vi "Main.vi"() -> ()   [LabVIEW 2021]
doc: "Use this template to build a simple state machine design pattern. Each state executes code and determines which state to transition to."
uses:
  controls/State.ctl
  controls/Data.ctl
  vmmultmso/vmmultmso.lvlib
panel:
  out "Device is OK?":bool
  out "Sample Rate 2":dbl
  out "Voltage Wave":dbl[][](graph)
  out "Device2 ID":dbl
  out "Sample Rate":dbl
  out "Device1 ID":dbl
  out "CH2 Min":dbl
  out "CH2 Max":dbl
  out "CH2 Vpp":dbl
  out "CH2 Frequency":dbl
  out "CH1 Frequency":dbl
  out "CH1 Vpp":dbl
  out "CH1 Max":dbl
  out "CH1 Min":dbl
  out "IO Read Return":u32 format="%x"
  out "IO4":bool
  out "IO0":bool
  out "Is IO Ready?":bool
  in  "DDS2 Amplitude":dbl=2000.0
  in  "DDS2 Bias":dbl
  in  "DDS2 Freq":dbl=1000.0
  in  "DDS2 Wave Style":u16(ring) items=["Sine", "Square", "Ramp"]
  in  "DDS1 Amplitude":dbl=2000.0
  in  "DDS1 Bias":dbl
  in  "DDS1 Freq":dbl=1000.0
  in  "DDS1 Wave Style":u16(ring) items=["Sine", "Square", "Ramp"]
  out "Is Data Ready？":bool
  out "ReadVoltageData Return":u32
  out "Voltage Wave":dbl[][](graph)
  out "Capture Return":i32
  out "Support Samples":u32[](array[numeric])
  in  "Exit":bool
  # "DDS1"
  # "DDS2"
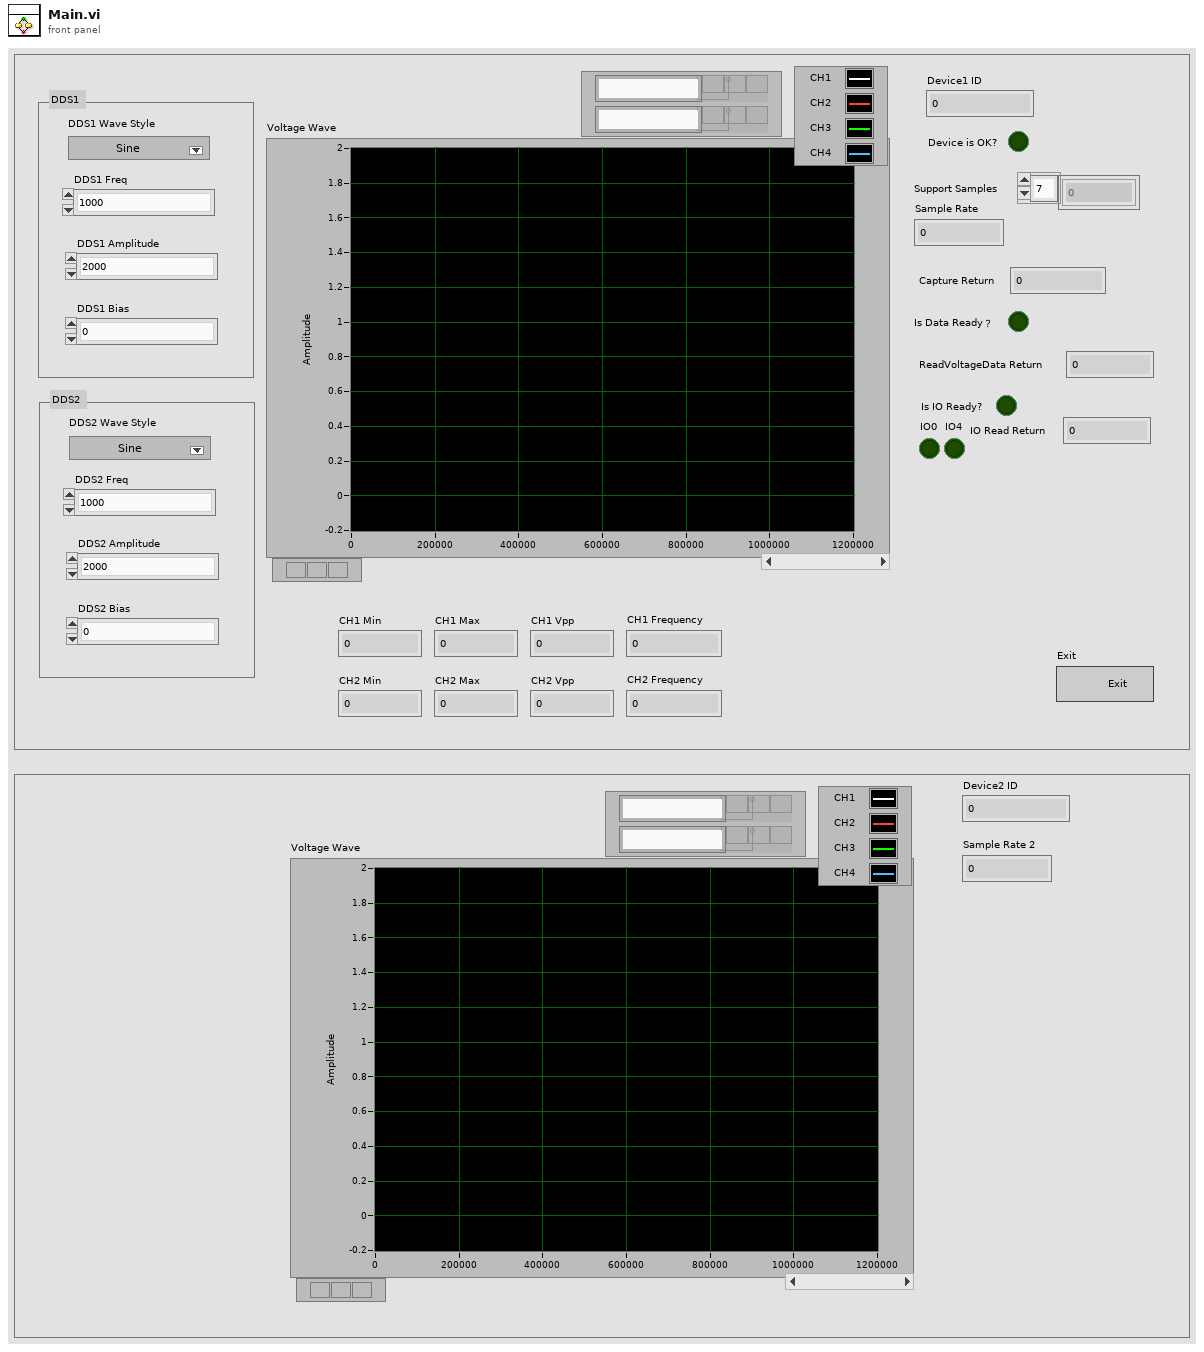
[diagram p1: front panel]
types:
  T1 = typedef "Data.ctl" = cluster{"Boolean <Is Exit>":bool, "String <Replace Me>":string, "Captue Length":dbl, "Device1 ID":dbl, "Device2 ID":dbl}
  T2 = typedef "State.ctl" = enum16{"Initialize", "Wait for UsbIn", "Init Osc and Dds", "Wait for Event", "Capture", "Read Voltage", "Read IO", "Exit"}
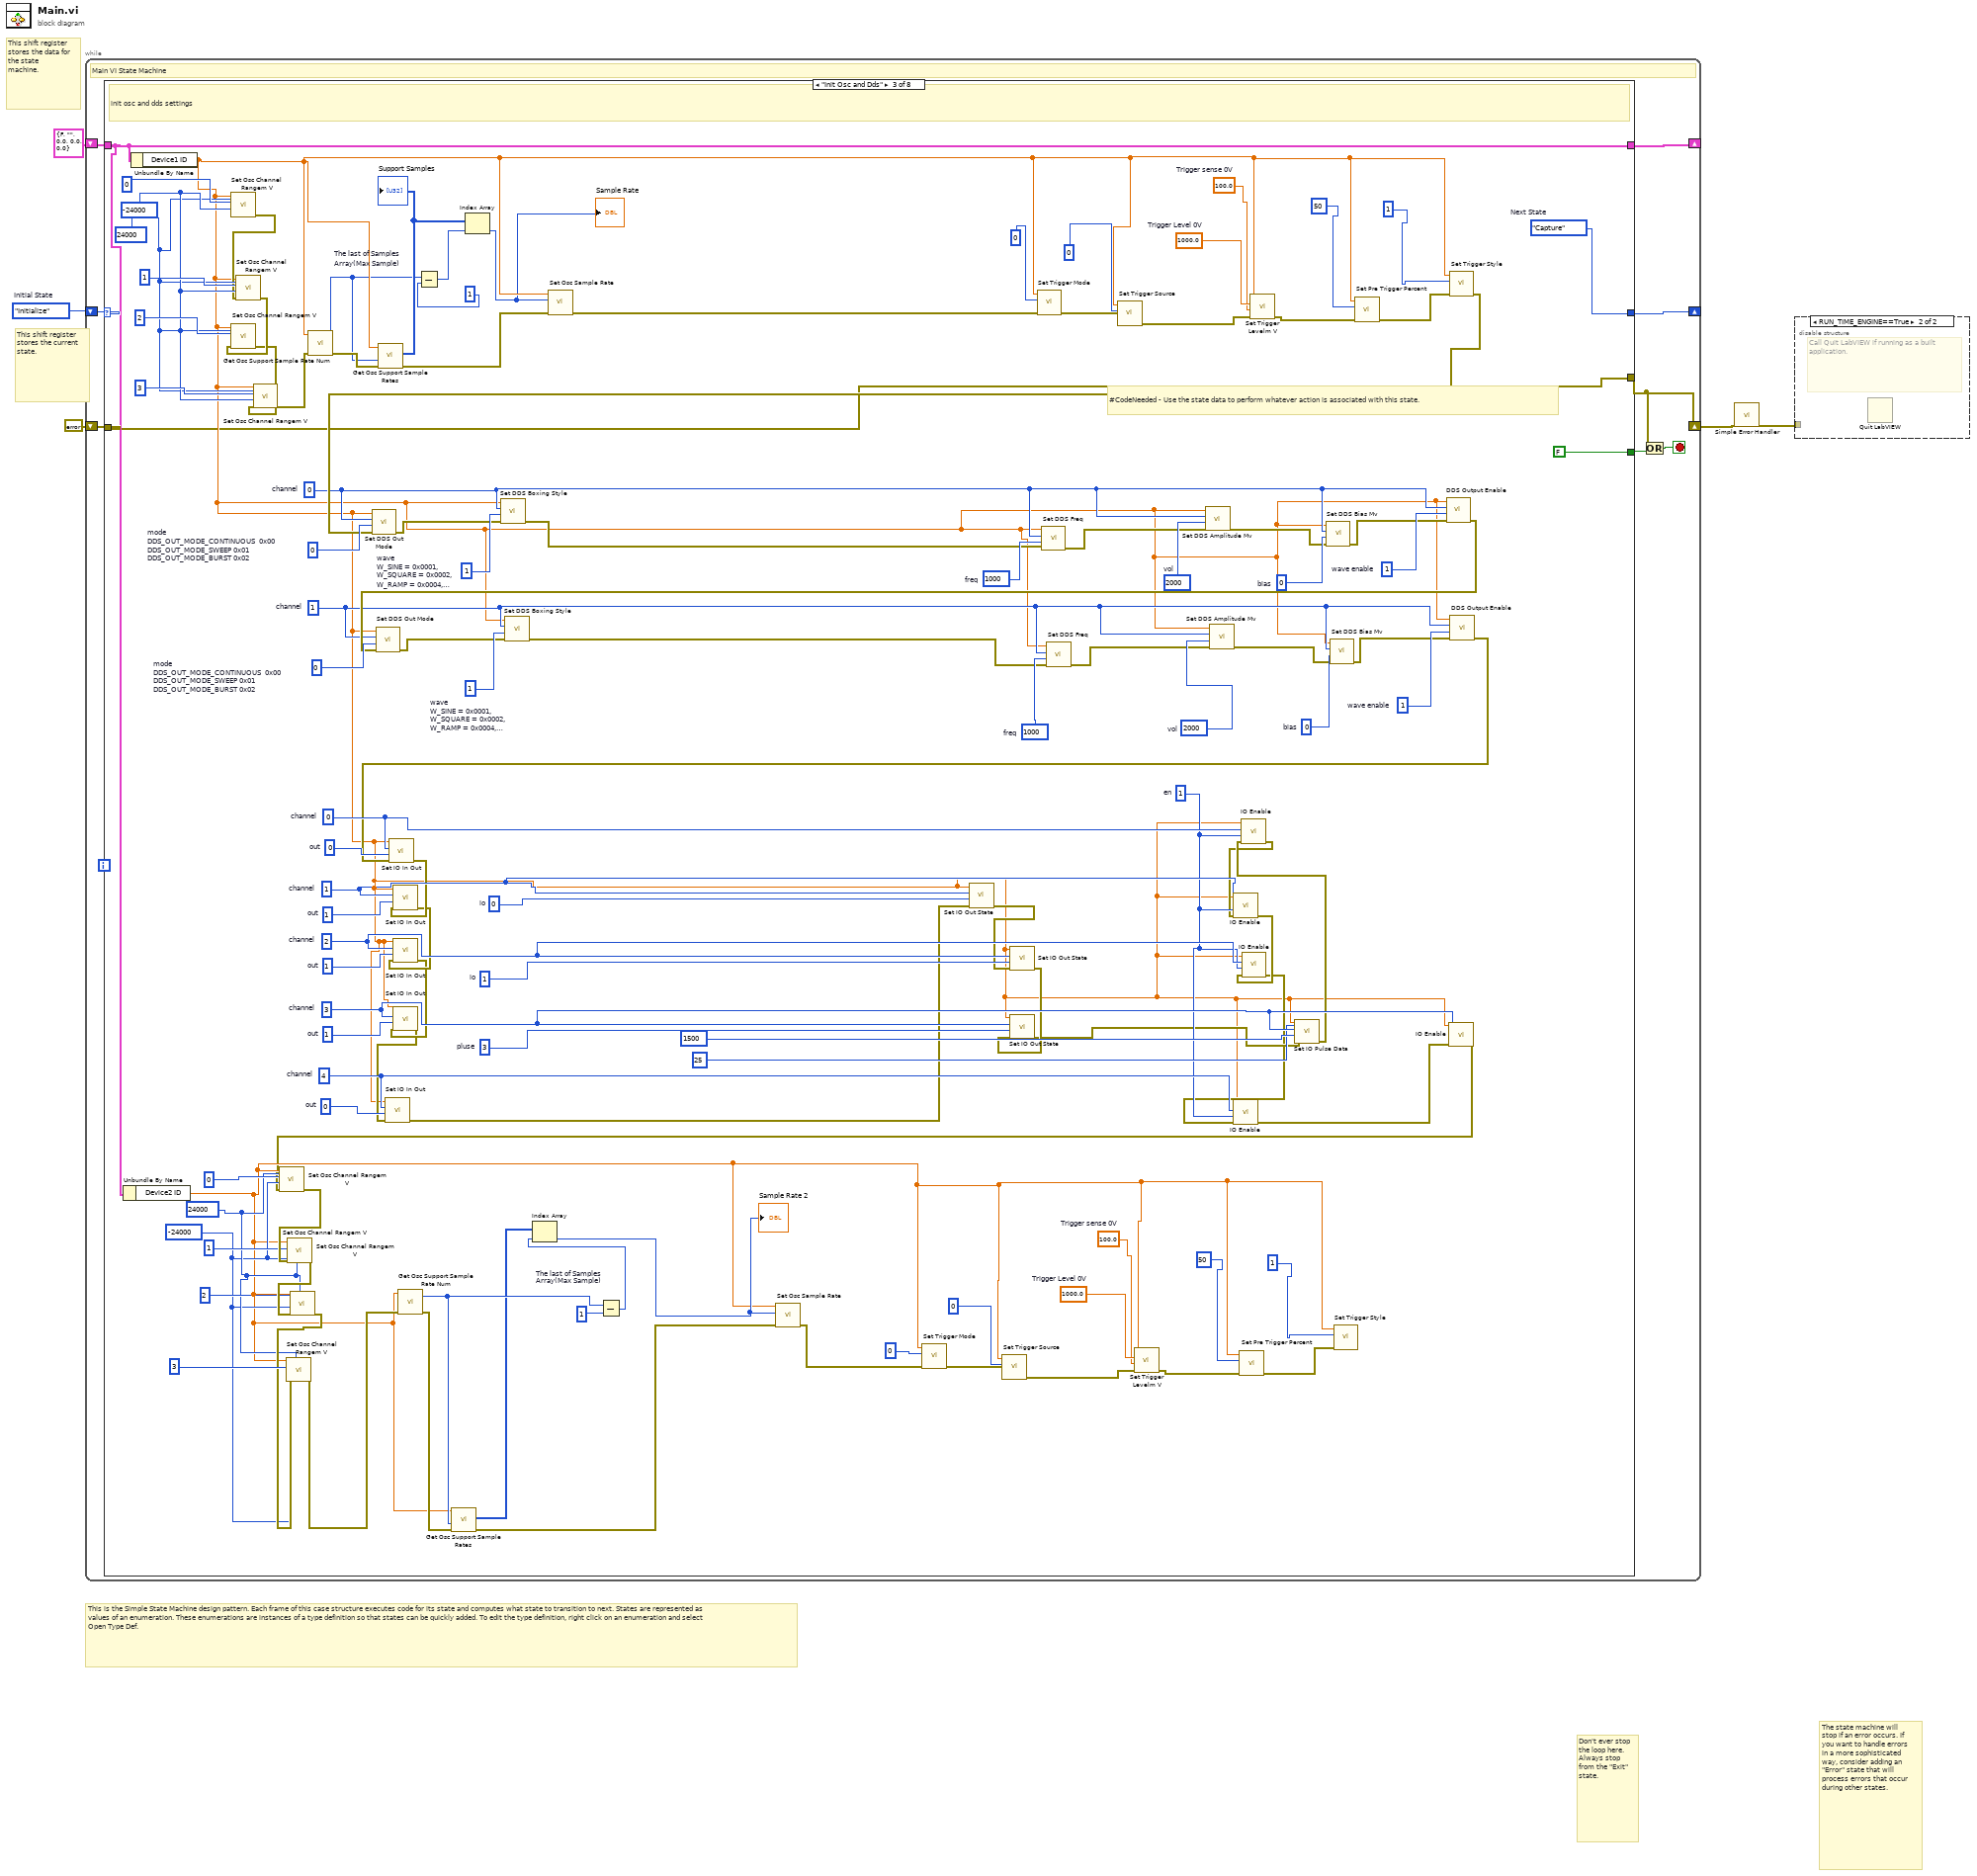
[diagram p0: block diagram]
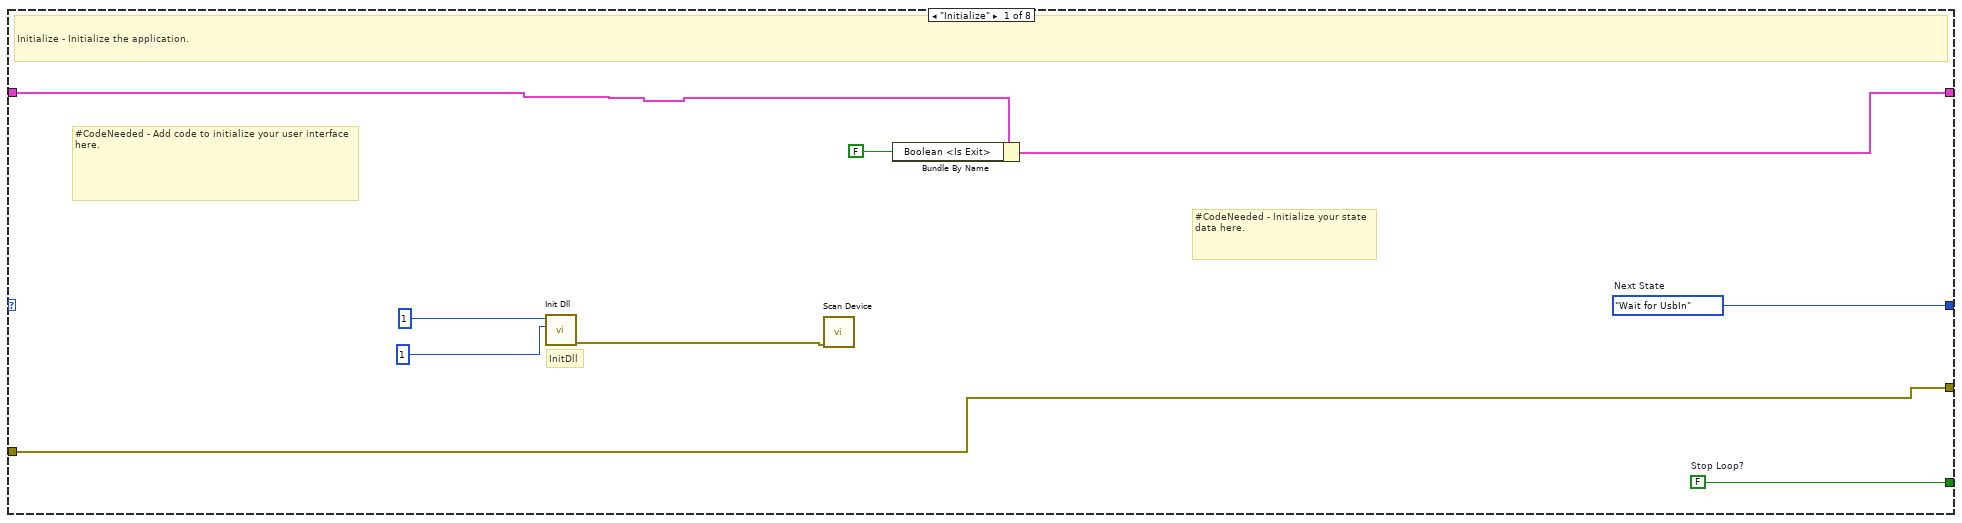
[diagram p3: hidden frame]
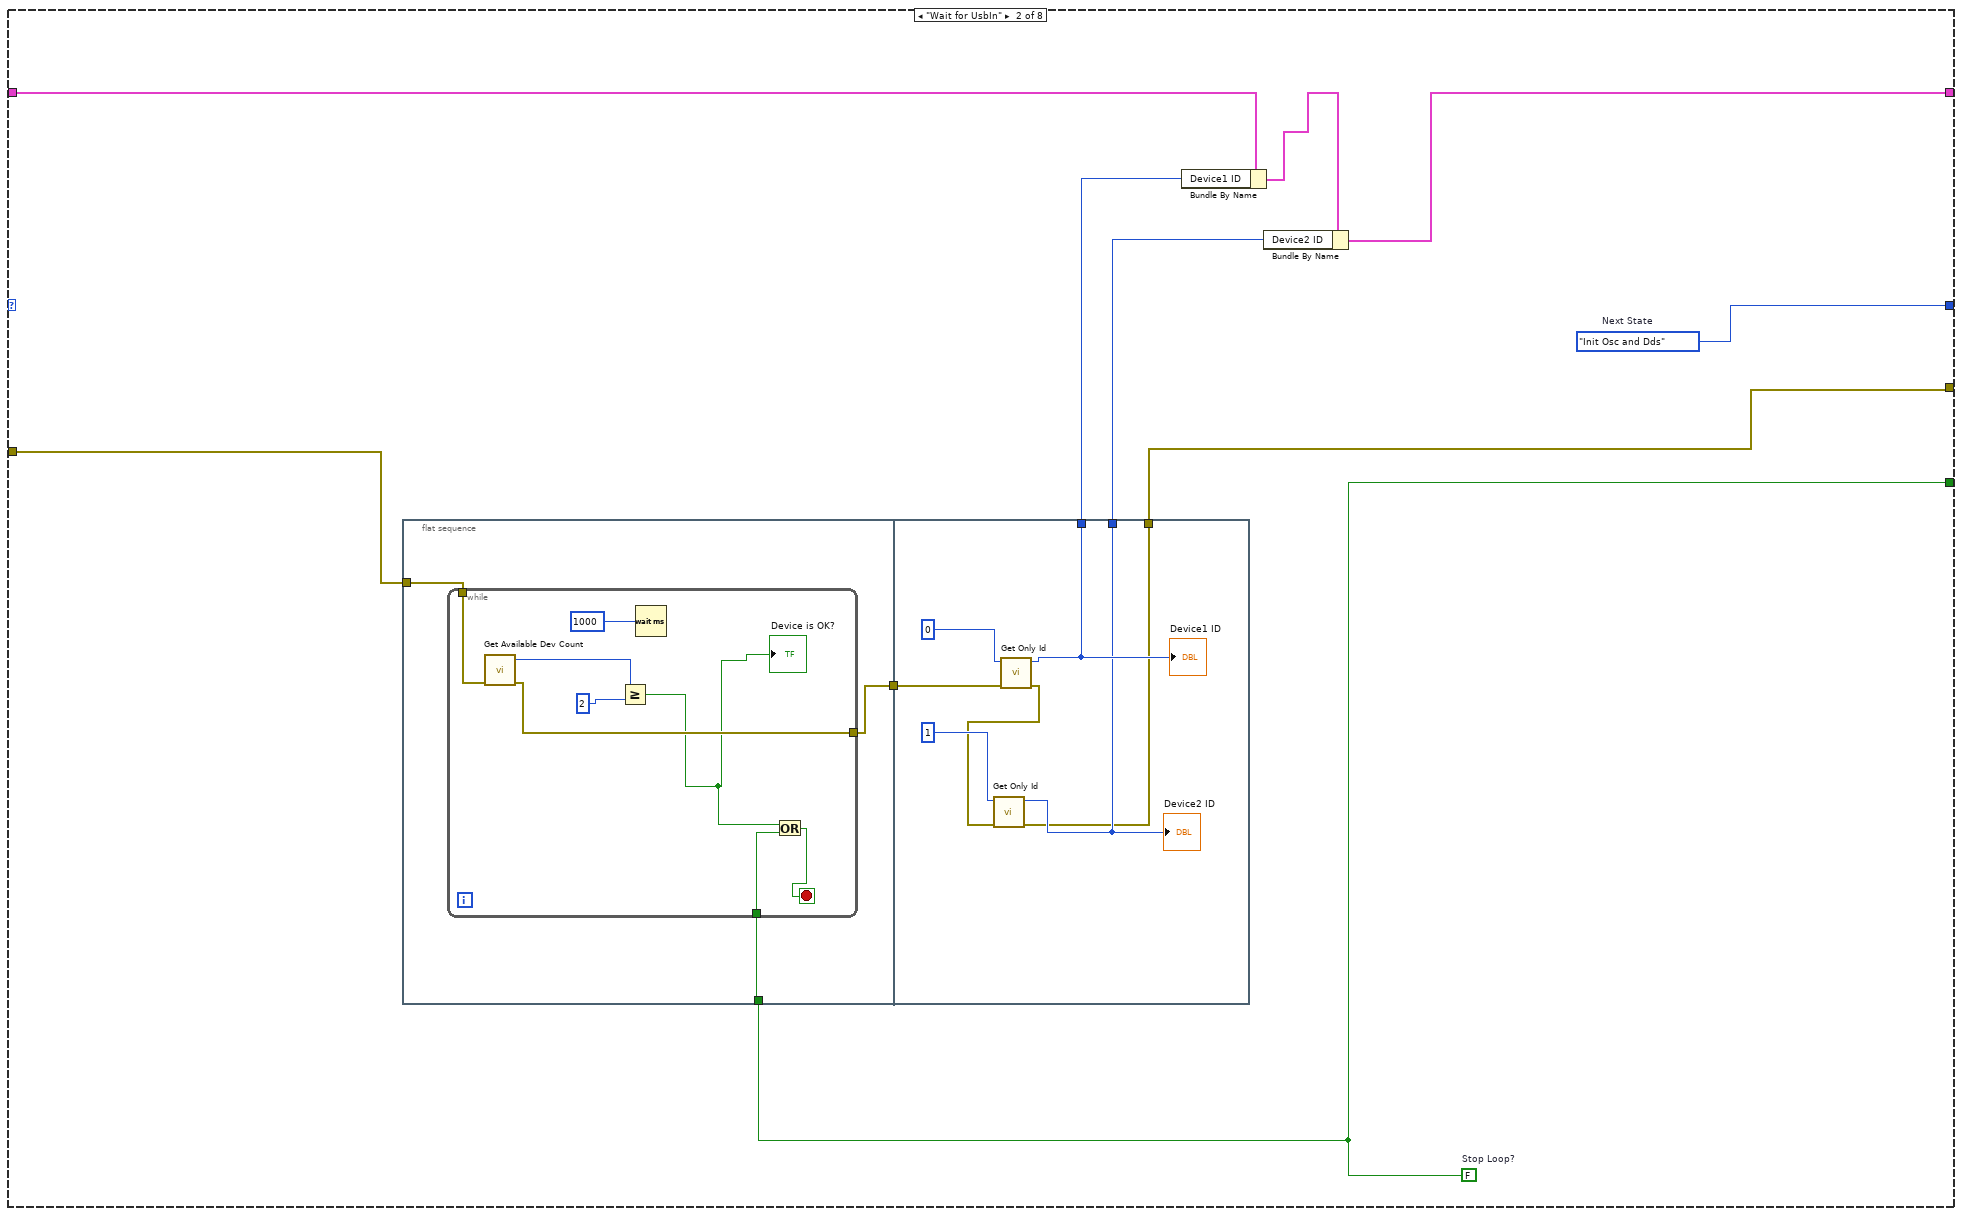
[diagram p4: hidden frame]
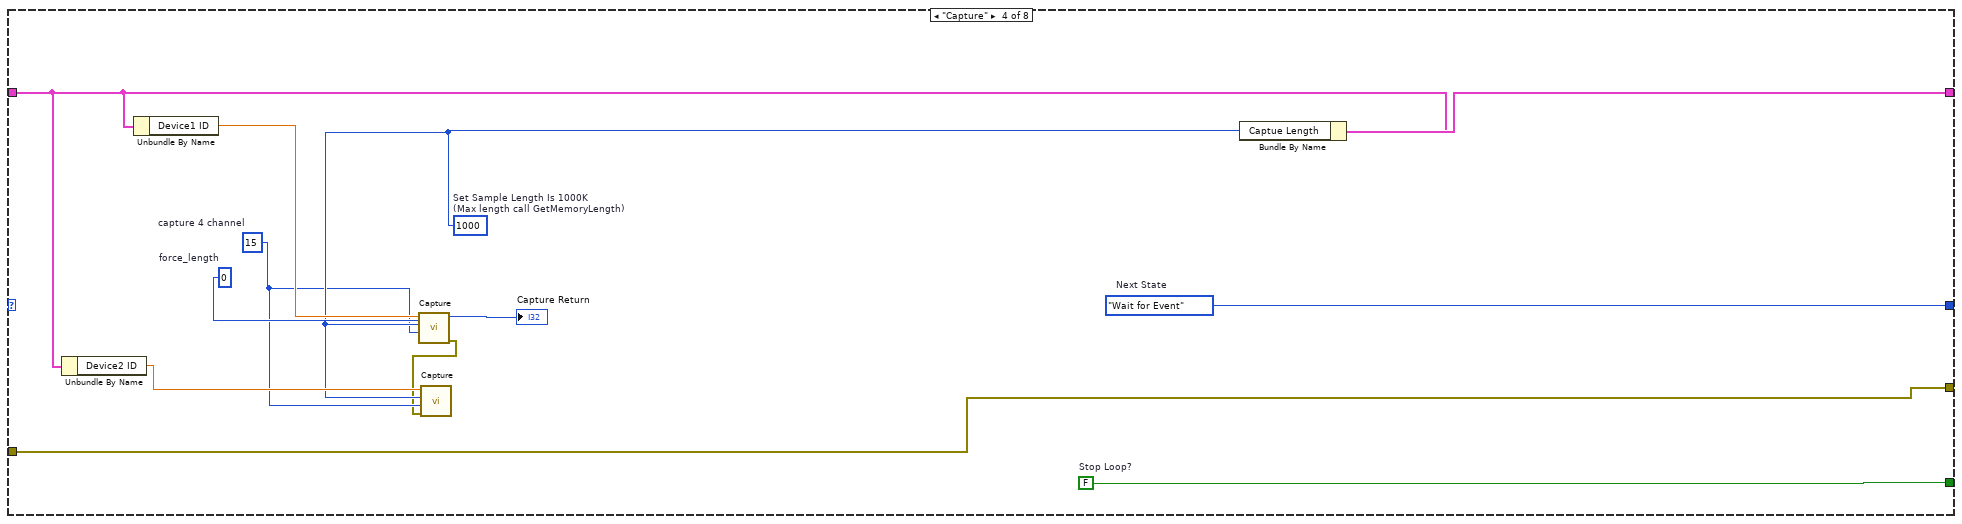
[diagram p5: hidden frame]
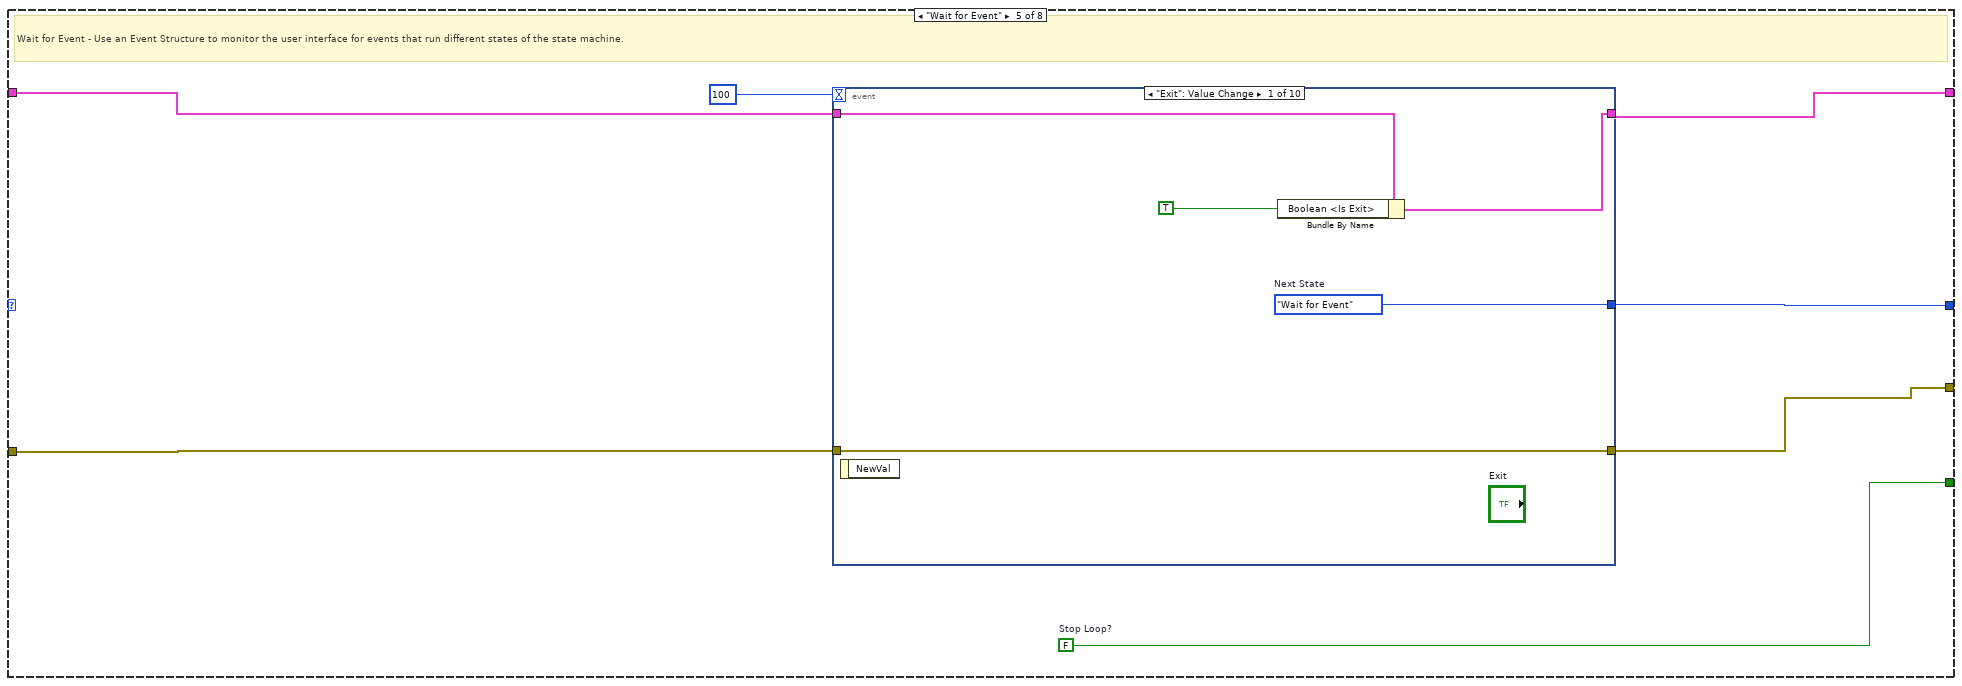
[diagram p6: hidden frame]
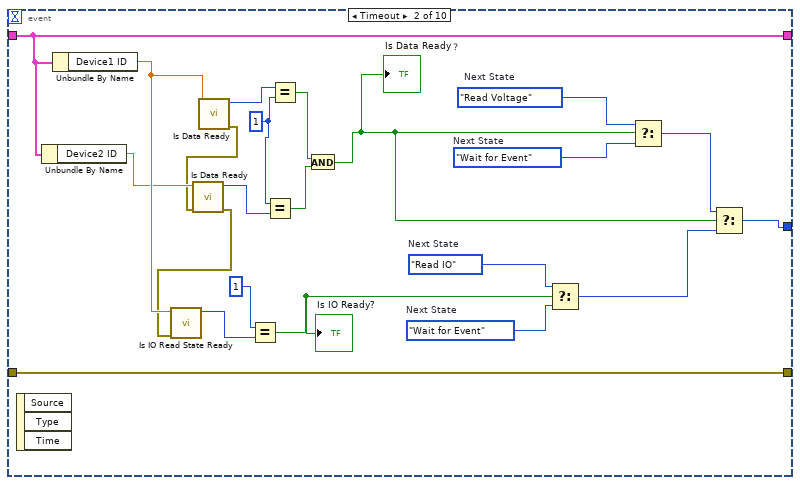
[diagram p7: hidden frame]
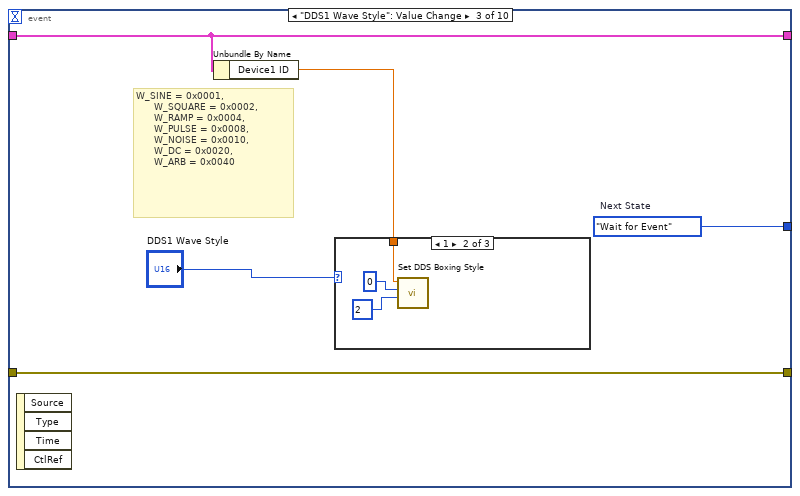
[diagram p8: hidden frame]
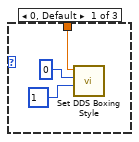
[diagram p9: hidden frame]
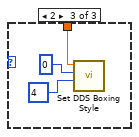
[diagram p10: hidden frame]
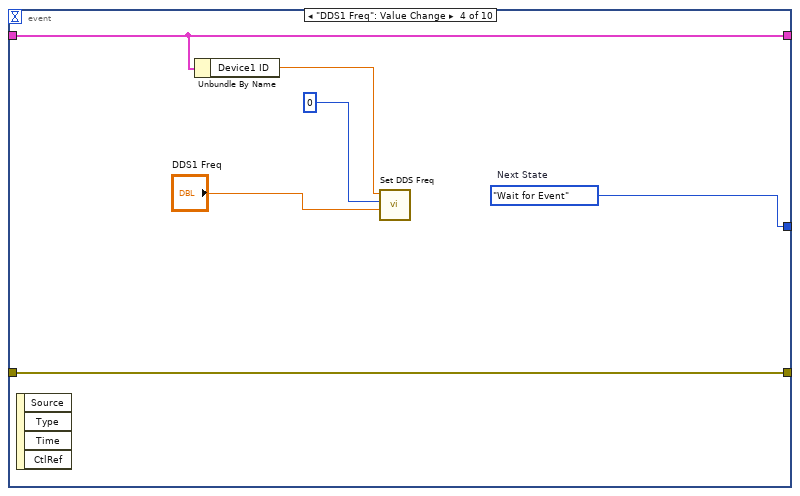
[diagram p11: hidden frame]
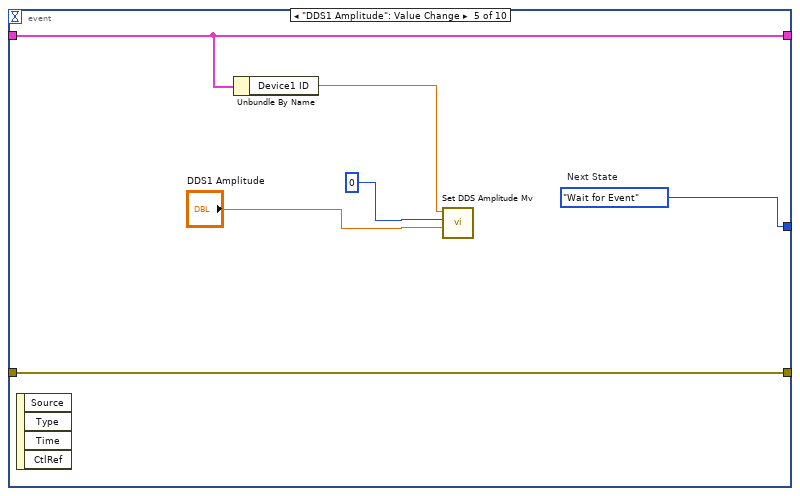
[diagram p12: hidden frame]
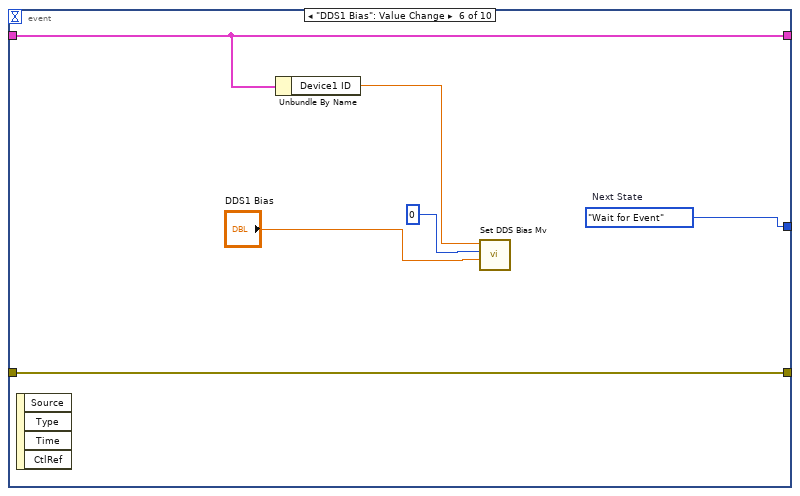
[diagram p13: hidden frame]
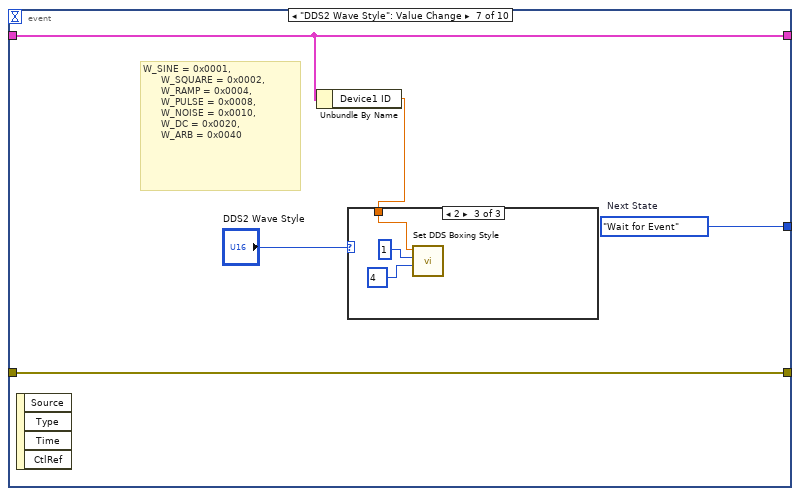
[diagram p14: hidden frame]
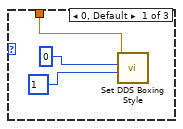
[diagram p15: hidden frame]
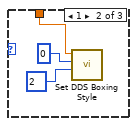
[diagram p16: hidden frame]
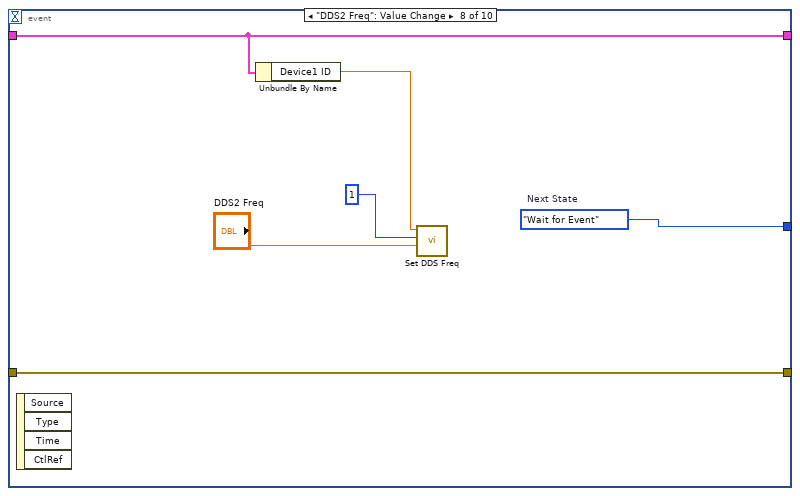
[diagram p17: hidden frame]
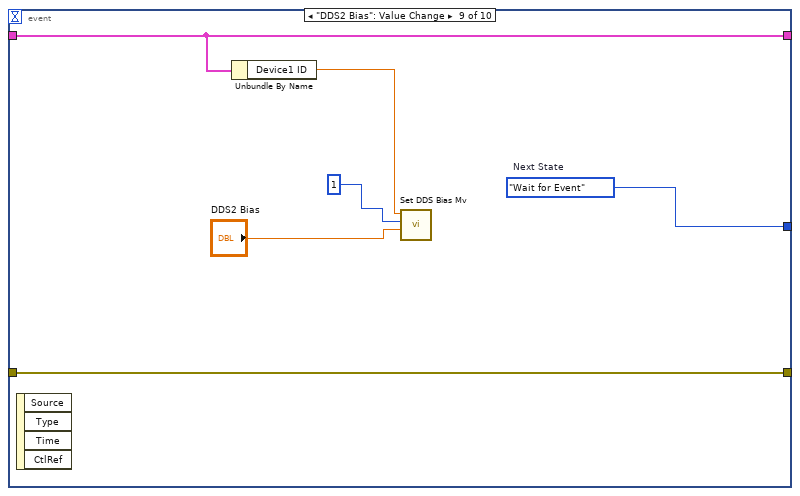
[diagram p18: hidden frame]
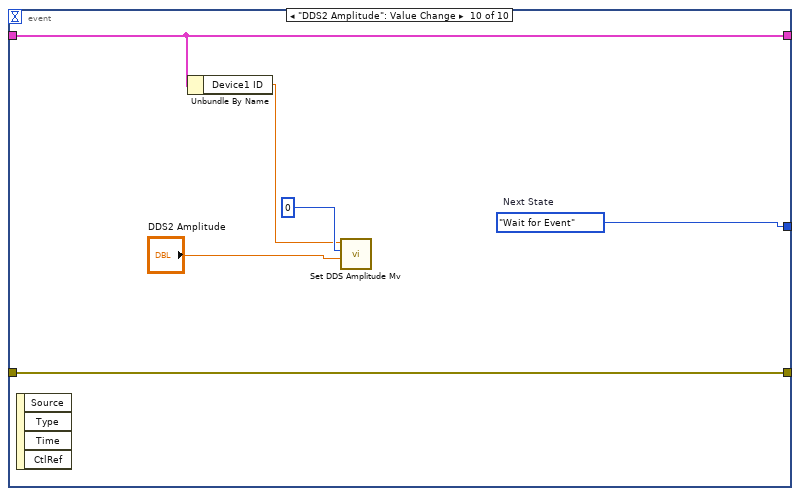
[diagram p19: hidden frame]
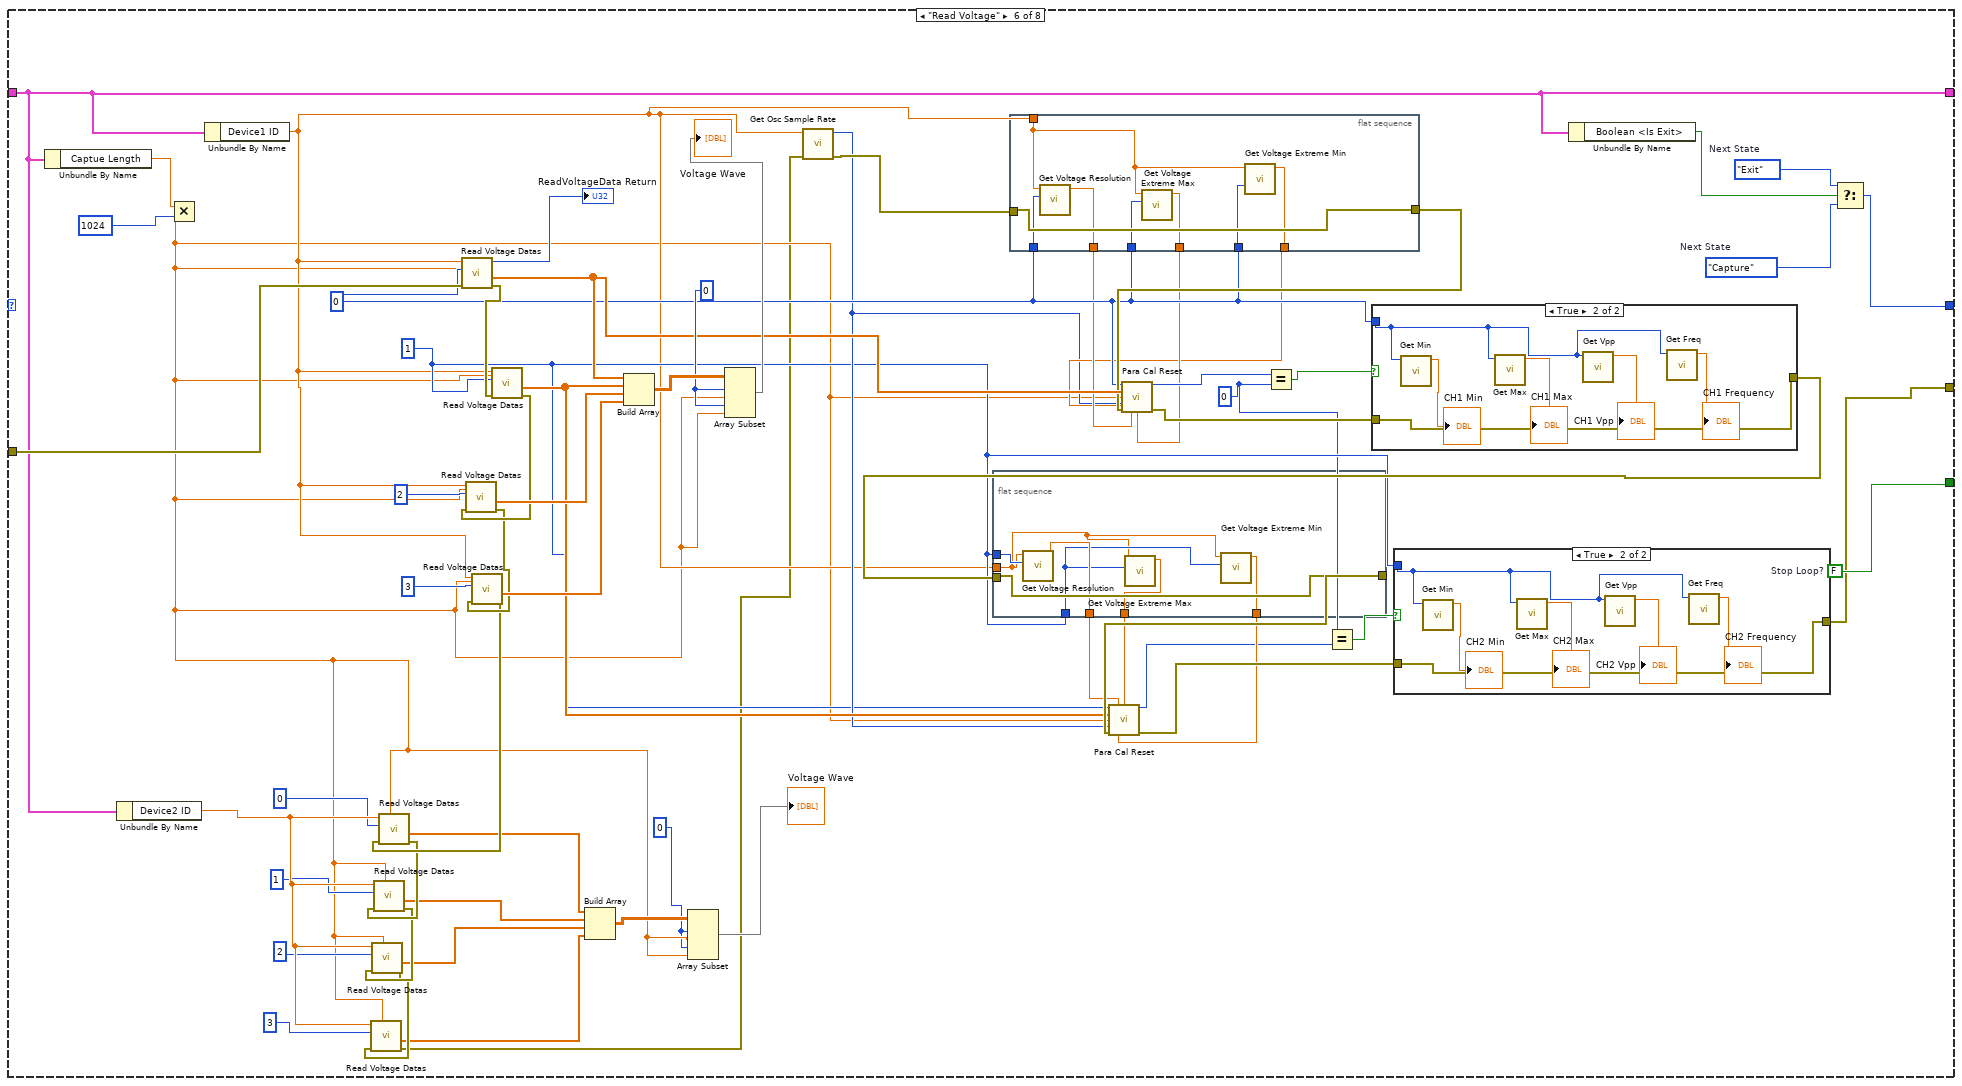
[diagram p20: hidden frame]
diagram:
  w5 = State."Initialize"  # Initial State
  # "Don't ever stop the loop here. Always stop from the \"Exit\" state."
  # "The state machine will stop if an error occurs. If you want to handle errors in a more sophisticated way, consider adding an \"Error\" state that will process errors that occur during other states."
  # "This shift register stores the data for the state machine."
  # "This is the Simple State Machine design pattern. Each frame of this case structure executes code for its state and computes what state to transition to next. States are represented as values of an enumeration. These enumerations are instances of a type definition so that states can be quickly added. To edit the type definition, right click on an enumeration and select Open Type Def."
  # "This shift register stores the current state."
  n1 = while {
    shift-right: [w12] -> _
    shift-left: w5 -> [w13]
    shift-right: [w10] -> _
    shift-left: T1 {"Boolean <Is Exit>"=FALSE, "String <Replace Me>"="", "Captue Length"=0.0, "Device1 ID"=0.0, "Device2 ID"=0.0} ("Data") -> [w11]
    shift-right: [w6] -> w2
    shift-left: errorcluster {"status"=FALSE, "code"=0, "source"=""} ("error constant") -> [w9]
    stop <- w8 stop-if-true
    # "Main VI State Machine"
    n2 = case shown="\"Init Osc and Dds\"" w13 {
      tunnel: [w22 w32 w169 w181 w188 w325 w375 w389] -> w12
      tunnel: w11 -> [w15 w25 w72 w175 w187 w299 w373 w386]
      tunnel: [w16 w26 w72 w177 w186 w299 w373 w386] -> w10
      tunnel: w9 -> [w14 w31 w51 w170 w185 w320 w371 w383]
      tunnel: [w21 w30 FALSE ("Stop Loop?") w180 w183 w341 w374 w388] -> w7
      tunnel: [w14 w23 w51 w170 w182 w280 w371 w383] -> w6
      frame "Initialize" {
        w21 = FALSE  # Stop Loop?
        w22 = State."Wait for UsbIn"  # Next State
        # "InitDll"
        # "#CodeNeeded - Initialize your state data here."
        # "#CodeNeeded - Add code to initialize your user interface here."
        # "Initialize - Initialize the application."
        n3 = call "Init Dll.vi"("en_hard_watchdog"=1 ("channel"), "en_log"=1 ("channel")) -> ("error out"=w18:errorcluster)  [unwired: 8 in, 1 out]
        n4 = call "Scan Device.vi"("error in (no error)"=w18) -> ()  [unwired: 9 in, 2 out]
        n5 = Bundle By Name(cluster=w15, "Boolean <Is Exit>"=FALSE) -> (w16:T1)
      }
      frame "Wait for UsbIn" {
        w32 = State."Init Osc and Dds"  # Next State
        w30 = FALSE  # Stop Loop?
        n6 = flat-sequence {
          tunnel: w31 -> [w35]
          tunnel: w30 -> [w34]
          tunnel: [w33] -> w29
          tunnel: w29 -> [w48]
          tunnel: [w46] -> w28
          tunnel: [w45] -> w27
          tunnel: [w44] -> w23
          frame #0 {
            n7 = while {
              tunnel: w34 -> [w42]
              tunnel: [w38] -> w33
              tunnel: w35 -> [w37]
              stop <- w41 stop-if-true
              n8 = call "Get Available Dev Count.vi"("error in (no error)"=w37) -> ("error out"=w38:errorcluster, "function return"=w40:i32)  [unwired: 9 in]
              n9 = Greater Or Equal?(x=w40, y=2 ("channel")) -> (x >= y?=w36:bool)
              "Device is OK?" <- w36
              n10 = Wait (ms)(milliseconds to wait=u32 1000 ("等待时间（毫秒）")) -> ()  [unwired: 1 out]
              n11 = Or(x=w36, y=w42) -> (x .or. y?=w41:bool)
            }
          }
          frame #1 {
            n12 = call "Get Only Id.vi"("error in (no error)"=w48, "dev_index"=0 ("channel")) -> ("error out"=w47:errorcluster, "function return"=w46:u32)  [unwired: 8 in]
            "Device1 ID" <- w46
            n13 = call "Get Only Id.vi"("error in (no error)"=w47, "dev_index"=1 ("channel")) -> ("error out"=w44:errorcluster, "function return"=w45:u32)  [unwired: 8 in]
            "Device2 ID" <- w45
          }
        }
        n14 = Bundle By Name(cluster=w25, "Device1 ID"=w28) -> (w24:T1)
        n15 = Bundle By Name(cluster=w24, "Device2 ID"=w27) -> (w26:T1)
      }
      frame "Init Osc and Dds" {
        w59 = sgl 100.0  # Trigger sense 0V
        w63 = sgl 1000.0  # Trigger Level 0V
        w69 = 24000 ("minmv")
        w68 = -24000 ("minmv")
        w130 = i8 0  # out
        w129 = i8 4  # channel
        w134 = i8 3  # pluse
        w135 = i8 1  # out
        w133 = i8 3  # channel
        w128 = i8 1  # en
        w139 = i8 0  # io
        w140 = i8 1  # io
        w141 = i8 1  # out
        w136 = i8 2  # channel
        w142 = i8 1  # out
        w137 = i8 1  # channel
        w143 = i8 0  # out
        w138 = i8 0  # channel
        w144 = sgl 100.0  # Trigger sense 0V
        w150 = i8 0  # mode DDS_OUT_MODE_CONTINUOUS  0x00 DDS_OUT_MODE_SWEEP 0x01 DDS_OUT_MODE_BURST 0x02
        w151 = i8 1  # wave enable
        w153 = u32 0  # bias
        w152 = u32 2000  # vol
        w89 = u32 1000  # freq
        w154 = i8 1  # wave  W_SINE = 0x0001,  W_SQUARE = 0x0002,  W_RAMP = 0x0004,  W_PULSE = 0x0008,  W_NOISE = 0x0010,  W_DC = 0x0020,  W_ARB = 0x0040
        w90 = i8 1  # channel
        w155 = i8 0  # mode DDS_OUT_MODE_CONTINUOUS  0x00 DDS_OUT_MODE_SWEEP 0x01 DDS_OUT_MODE_BURST 0x02
        w156 = i8 1  # wave enable
        w158 = u32 0  # bias
        w157 = u32 2000  # vol
        w93 = u32 1000  # freq
        w159 = i8 1  # wave  W_SINE = 0x0001,  W_SQUARE = 0x0002,  W_RAMP = 0x0004,  W_PULSE = 0x0008,  W_NOISE = 0x0010,  W_DC = 0x0020,  W_ARB = 0x0040
        w94 = i8 0  # channel
        w165 = sgl 1000.0  # Trigger Level 0V
        w145 = 24000 ("minmv")
        w146 = -24000 ("minmv")
        w169 = State."Capture"  # Next State
        # "#CodeNeeded - Use the state data to perform whatever action is associated with this state."
        # "init osc and dds settings"
        n16 = Unbundle By Name(w72) -> ("Device2 ID"=w54:dbl)
        n17 = Unbundle By Name(w72) -> ("Device1 ID"=w86:dbl)
        n18 = call "Set Osc Channel Rangem V.vi"("maxmv"=w145, "minmv"=w146, "channel"=0, "dev_id"=w86) -> ("error out"=w127:errorcluster)  [unwired: 6 in, 1 out]
        n19 = call "Set Osc Channel Rangem V.vi"("maxmv"=w145, "error in (no error)"=w127, "minmv"=w146, "channel"=1, "dev_id"=w86) -> ("error out"=w126:errorcluster)  [unwired: 5 in, 1 out]
        n20 = call "Set Osc Channel Rangem V.vi"("maxmv"=w145, "error in (no error)"=w126, "minmv"=w146, "channel"=2, "dev_id"=w86) -> ("error out"=w125:errorcluster)  [unwired: 5 in, 1 out]
        n21 = call "Set Osc Channel Rangem V.vi"("maxmv"=w145, "error in (no error)"=w125, "minmv"=w146, "channel"=3, "dev_id"=w86) -> ("error out"=w124:errorcluster)  [unwired: 5 in, 1 out]
        n22 = call "Get Osc Support Sample Rate Num.vi"("error in (no error)"=w124, "dev_id"=w86) -> ("error out"=w123:errorcluster, "function return"=w84:i32)  [unwired: 8 in]
        n23 = call "Get Osc Support Sample Rates.vi"("error in (no error)"=w123, "maxnum"=w84, "dev_id"=w86) -> ("error out"=w122:errorcluster, "sample out"=w161:u32[])  [unwired: 6 in, 1 out]
        "Support Samples" <- w161
        n24 = Subtract "The last of Samples Array(Max Sample)"(x=w84, y=1 ("front")) -> (x-y=w83:i32)
        n25 = Index Array(array=w161, index=w83) -> (element=w85:u32)
        "Sample Rate" <- w85
        n26 = call "Set Osc Sample Rate.vi"("error in (no error)"=w122, "sample"=w85, "dev_id"=w86) -> ("error out"=w121:errorcluster)  [unwired: 7 in, 1 out]
        n27 = call "Set Trigger Mode.vi"("error in (no error)"=w121, "mode"=0 ("front"), "dev_id"=w86) -> ("error out"=w120:errorcluster)  [unwired: 8 in]
        n28 = call "Set Trigger Source.vi"("error in (no error)"=w120, "source"=0 ("front"), "dev_id"=w86) -> ("error out"=w119:errorcluster)  [unwired: 8 in]
        n29 = call "Set Trigger Levelm V.vi"("error in (no error)"=w119, "sense_mv"=w144, "level_mv"=w165, "dev_id"=w86) -> ("error out"=w118:errorcluster)  [unwired: 7 in]
        n30 = call "Set Pre Trigger Percent.vi"("error in (no error)"=w118, "front"=50, "dev_id"=w86) -> ("error out"=w117:errorcluster)  [unwired: 8 in]
        n31 = call "Set Trigger Style.vi"("error in (no error)"=w117, "style"=u32 1, "dev_id"=w86) -> ("error out"=w116:errorcluster)  [unwired: 8 in]
        n32 = call "Set DDS Out Mode.vi"("error in (no error)"=w116, "out_mode"=w155, "channel_index"=w94, "dev_id"=w86) -> ("error out"=w115:errorcluster)  [unwired: 7 in]
        n33 = call "Set DDS Boxing Style.vi"("error in (no error)"=w115, "boxing"=w159, "channel_index"=w94, "dev_id"=w86) -> ("error out"=w92:errorcluster)  [unwired: 7 in]
        n34 = call "Set DDS Freq.vi"("error in (no error)"=w92, "freq"=w93, "channel_index"=w94, "dev_id"=w86) -> ("error out"=w91:errorcluster)  [unwired: 7 in]
        n35 = call "Set DDS Amplitude Mv.vi"("error in (no error)"=w91, "amplitdude"=w157, "channel_index"=w94, "dev_id"=w86) -> ("error out"=w114:errorcluster)  [unwired: 7 in]
        n36 = call "Set DDS Bias Mv.vi"("error in (no error)"=w114, "bias"=w158, "channel_index"=w94, "dev_id"=w86) -> ("error out"=w113:errorcluster)  [unwired: 7 in]
        n37 = call "DDS Output Enable.vi"("error in (no error)"=w113, "enable"=w156, "channel_index"=w94, "dev_id"=w86) -> ("error out"=w112:errorcluster)  [unwired: 7 in]
        n38 = call "Set DDS Out Mode.vi"("error in (no error)"=w112, "out_mode"=w150, "channel_index"=w90, "dev_id"=w86) -> ("error out"=w111:errorcluster)  [unwired: 7 in]
        n39 = call "Set DDS Boxing Style.vi"("error in (no error)"=w111, "boxing"=w154, "channel_index"=w90, "dev_id"=w86) -> ("error out"=w88:errorcluster)  [unwired: 7 in]
        n40 = call "Set DDS Freq.vi"("error in (no error)"=w88, "freq"=w89, "channel_index"=w90, "dev_id"=w86) -> ("error out"=w87:errorcluster)  [unwired: 7 in]
        n41 = call "Set DDS Amplitude Mv.vi"("error in (no error)"=w87, "amplitdude"=w152, "channel_index"=w90, "dev_id"=w86) -> ("error out"=w110:errorcluster)  [unwired: 7 in]
        n42 = call "Set DDS Bias Mv.vi"("error in (no error)"=w110, "bias"=w153, "channel_index"=w90, "dev_id"=w86) -> ("error out"=w109:errorcluster)  [unwired: 7 in]
        n43 = call "DDS Output Enable.vi"("error in (no error)"=w109, "enable"=w151, "channel_index"=w90, "dev_id"=w86) -> ("error out"=w108:errorcluster)  [unwired: 7 in]
        n44 = call "Set IO In Out.vi"("error in (no error)"=w108, "inout"=w143, "channel"=w138, "dev_id"=w86) -> ("error out"=w107:errorcluster)  [unwired: 7 in]
        n45 = call "Set IO In Out.vi"("error in (no error)"=w107, "inout"=w142, "channel"=w137, "dev_id"=w86) -> ("error out"=w106:errorcluster)  [unwired: 7 in]
        n46 = call "Set IO In Out.vi"("error in (no error)"=w106, "inout"=w141, "channel"=w136, "dev_id"=w86) -> ("error out"=w105:errorcluster)  [unwired: 7 in]
        n47 = call "Set IO In Out.vi"("error in (no error)"=w105, "inout"=w135, "channel"=w133, "dev_id"=w86) -> ("error out"=w104:errorcluster)  [unwired: 7 in]
        n48 = call "Set IO In Out.vi"("error in (no error)"=w104, "inout"=w130, "channel"=w129, "dev_id"=w86) -> ("error out"=w103:errorcluster)  [unwired: 7 in]
        n49 = call "Set IO Out State.vi"("error in (no error)"=w103, "state"=w139, "channel"=w137, "dev_id"=w86) -> ("error out"=w102:errorcluster)  [unwired: 7 in]
        n50 = call "Set IO Out State.vi"("error in (no error)"=w102, "state"=w140, "channel"=w136, "dev_id"=w86) -> ("error out"=w101:errorcluster)  [unwired: 7 in]
        n51 = call "Set IO Out State.vi"("error in (no error)"=w101, "state"=w134, "channel"=w133, "dev_id"=w86) -> ("error out"=w100:errorcluster)  [unwired: 7 in]
        n52 = call "Set IO Pulse Data.vi"("duty"=25 ("minmv"), "error in (no error)"=w100, "hz"=1500 ("minmv"), "channel"=w133, "dev_id"=w86) -> ("error out"=w99:errorcluster)  [unwired: 6 in]
        n53 = call "IO Enable.vi"("error in (no error)"=w99, "enable"=w128, "channel"=w138, "dev_id"=w86) -> ("error out"=w98:errorcluster)  [unwired: 7 in]
        n54 = call "IO Enable.vi"("error in (no error)"=w98, "enable"=w128, "channel"=w137, "dev_id"=w86) -> ("error out"=w97:errorcluster)  [unwired: 7 in]
        n55 = call "IO Enable.vi"("error in (no error)"=w97, "enable"=w128, "channel"=w136, "dev_id"=w86) -> ("error out"=w96:errorcluster)  [unwired: 7 in]
        n56 = call "IO Enable.vi"("error in (no error)"=w96, "enable"=w128, "channel"=w129, "dev_id"=w86) -> ("error out"=w95:errorcluster)  [unwired: 7 in]
        n57 = call "IO Enable.vi"("error in (no error)"=w95, "channel"=w133, "dev_id"=w86) -> ("error out"=w52:errorcluster)  [unwired: 8 in]
        n58 = call "Set Osc Channel Rangem V.vi"("maxmv"=w69, "error in (no error)"=w52, "minmv"=w68, "channel"=0, "dev_id"=w54) -> ("error out"=w78:errorcluster)  [unwired: 5 in, 1 out]
        n59 = call "Set Osc Channel Rangem V.vi"("maxmv"=w69, "error in (no error)"=w78, "minmv"=w68, "channel"=1, "dev_id"=w54) -> ("error out"=w79:errorcluster)  [unwired: 5 in, 1 out]
        n60 = call "Set Osc Channel Rangem V.vi"("maxmv"=w69, "error in (no error)"=w79, "minmv"=w68, "channel"=2, "dev_id"=w54) -> ("error out"=w70:errorcluster)  [unwired: 5 in, 1 out]
        n61 = call "Set Osc Channel Rangem V.vi"("maxmv"=w69, "error in (no error)"=w70, "minmv"=w68, "channel"=3, "dev_id"=w54) -> ("error out"=w67:errorcluster)  [unwired: 5 in, 1 out]
        n62 = call "Get Osc Support Sample Rate Num.vi"("error in (no error)"=w67, "dev_id"=w54) -> ("error out"=w66:errorcluster, "function return"=w81:i32)  [unwired: 8 in]
        n63 = call "Get Osc Support Sample Rates.vi"("error in (no error)"=w66, "maxnum"=w81, "dev_id"=w54) -> ("error out"=w65:errorcluster, "sample out"=w77:u32[])  [unwired: 6 in, 1 out]
        n64 = Subtract "The last of Samples Array(Max Sample)"(x=w81, y=1 ("front")) -> (x-y=w82:i32)
        n65 = Index Array(array=w77, index=w82) -> (element=w80:u32)
        "Sample Rate 2" <- w80
        n66 = call "Set Osc Sample Rate.vi"("error in (no error)"=w65, "sample"=w80, "dev_id"=w54) -> ("error out"=w53:errorcluster)  [unwired: 7 in, 1 out]
        n67 = call "Set Trigger Mode.vi"("error in (no error)"=w53, "mode"=0 ("front"), "dev_id"=w54) -> ("error out"=w58:errorcluster)  [unwired: 8 in]
        n68 = call "Set Trigger Source.vi"("error in (no error)"=w58, "source"=0 ("front"), "dev_id"=w54) -> ("error out"=w57:errorcluster)  [unwired: 8 in]
        n69 = call "Set Trigger Levelm V.vi"("error in (no error)"=w57, "sense_mv"=w59, "level_mv"=w63, "dev_id"=w54) -> ("error out"=w56:errorcluster)  [unwired: 7 in]
        n70 = call "Set Pre Trigger Percent.vi"("error in (no error)"=w56, "front"=50, "dev_id"=w54) -> ("error out"=w55:errorcluster)  [unwired: 8 in]
        n71 = call "Set Trigger Style.vi"("error in (no error)"=w55, "style"=u32 1, "dev_id"=w54) -> ()  [unwired: 8 in, 1 out]
      }
      frame "Capture" {
        w178 = i8 0  # force_length
        w173 = u32 1000  # Set Sample Length Is 1000K (Max length call GetMemoryLength)
        w172 = i8 15  # capture 4 channel
        w180 = FALSE  # Stop Loop?
        w181 = State."Wait for Event"  # Next State
        n72 = Unbundle By Name(w175) -> ("Device2 ID"=w174:dbl)
        n73 = Unbundle By Name(w175) -> ("Device1 ID"=w176:dbl)
        n74 = call "Capture.vi"("force_length"=w178, "capture_channel"=w172, "length"=w173, "dev_id"=w176) -> ("error out"=w171:errorcluster, "function return"=→"Capture Return":i32)  [unwired: 6 in]
        n75 = call "Capture.vi"("error in (no error)"=w171, "capture_channel"=w172, "length"=w173, "dev_id"=w174) -> ()  [unwired: 6 in, 2 out]
        n76 = Bundle By Name(cluster=w175, "Captue Length"=w173) -> (w177:T1)
      }
      frame "Wait for Event" {
        w183 = FALSE  # Stop Loop?
        # "Wait for Event - Use an Event Structure to monitor the user interface for events that run different states of the state machine."
        n77 = event shown="[0] \"Exit\": Value Change" {
          selector: _ -> [_ _ _ _ _ _ _ _ _ _]
          dyn-events: _ -> [_ _ _ _ _ _ _ _ _ _]
          timeout: 100 ("y") -> [_ _ _ _ _ _ _ _ _ _]
          tunnel: [w193 w205 w218 w234 w240 w246 w251 w266 w271 w277] -> w188
          tunnel: w187 -> [w190 w202 w217 w230 w237 w243 w249 w263 w269 w274]
          tunnel: [w189 w202 w217 w230 w237 w243 w249 w263 w269 w274] -> w186
          tunnel: w185 -> [w192 w215 w220 w235 w241 w247 w252 w267 w273 w279]
          tunnel: [w192 w215 w220 w235 w241 w247 w252 w267 w273 w279] -> w182
          event "Exit": Value Change {
            w193 = State."Wait for Event"  # Next State
            n78 = event-data() -> ()  [unwired: 1 in, 1 out]
            n79 = Bundle By Name(cluster=w190, "Boolean <Is Exit>"=TRUE) -> (w189:T1)
          }
          event Timeout {
            w209 = State."Wait for Event"  # Next State
            w210 = State."Read IO"  # Next State
            w212 = State."Wait for Event"  # Next State
            w200 = 1 ("y")
            w213 = State."Read Voltage"  # Next State
            n80 = event-data() -> ()  [unwired: 1 in, 3 out]
            n81 = Unbundle By Name(w202) -> ("Device2 ID"=w201:dbl)
            n82 = Unbundle By Name(w202) -> ("Device1 ID"=w203:dbl)
            n83 = call "Is Data Ready.vi"("dev_id"=w203) -> ("error out"=w198:errorcluster, "function return"=w214:i32)  [unwired: 9 in]
            n84 = call "Is Data Ready.vi"("error in (no error)"=w198, "dev_id"=w201) -> ("error out"=w197:errorcluster, "function return"=w199:i32)  [unwired: 8 in]
            n85 = call "Is IO Read State Ready.vi"("error in (no error)"=w197, "dev_id"=w203) -> ("function return"=w204:i32)  [unwired: 8 in, 1 out]
            n86 = Equal?(x=1 ("y"), y=w204) -> (x = y?=w211:bool)
            "Is IO Ready?" <- w211
            n87 = Equal?(x=w200, y=w199) -> (x = y?=w196:bool)
            n88 = Equal?(x=w214, y=w200) -> (x = y?=w195:bool)
            n89 = And(x=w195, y=w196) -> (x .and. y?=w194:bool)
            "Is Data Ready？" <- w194
            n90 = Select(t=w210, s=w211, f=w209) -> (s? t:f=w207:T2)
            n91 = Select(t=w213, s=w194, f=w212) -> (s? t:f=w206:T2)
            n92 = Select(t=w206, s=w194, f=w207) -> (s? t:f=w205:T2)
          }
          event "DDS1 Wave Style": Value Change {
            w218 = State."Wait for Event"  # Next State
            # "W_SINE = 0x0001, \n\t\t\t\t\t\tW_SQUARE = 0x0002, \n\t\t\t\t\t\tW_RAMP = 0x0004, \n\t\t\t\t\t\tW_PULSE = 0x0008, \n\t\t\t\t\t\tW_NOISE = 0x0010, \n\t\t\t\t\t\tW_DC = 0x0020, \n\t\t\t\t\t\tW_ARB = 0x0040"
            n93 = event-data() -> ()  [unwired: 1 in, 4 out]
            n94 = Unbundle By Name(w217) -> ("Device1 ID"=w216:dbl)
            n95 = case shown="1" "DDS1 Wave Style" {
              tunnel: w216 -> [w221 w224 w227]
              frame 0, Default {
                n96 = call "Set DDS Boxing Style.vi"("boxing"=1 ("y"), "channel_index"=0 ("y"), "dev_id"=w221) -> ()  [unwired: 8 in, 1 out]
              }
              frame 1 {
                n97 = call "Set DDS Boxing Style.vi"("boxing"=2 ("y"), "channel_index"=0 ("y"), "dev_id"=w224) -> ()  [unwired: 8 in, 1 out]
              }
              frame 2 {
                n98 = call "Set DDS Boxing Style.vi"("boxing"=4 ("y"), "channel_index"=0 ("y"), "dev_id"=w227) -> ()  [unwired: 8 in, 1 out]
              }
            }
          }
          event "DDS1 Freq": Value Change {
            w234 = State."Wait for Event"  # Next State
            n99 = event-data() -> ()  [unwired: 1 in, 4 out]
            n100 = Unbundle By Name(w230) -> ("Device1 ID"=w231:dbl)
            n101 = call "Set DDS Freq.vi"("freq"="DDS1 Freq", "channel_index"=0 ("y"), "dev_id"=w231) -> ()  [unwired: 8 in, 1 out]
          }
          event "DDS1 Amplitude": Value Change {
            w240 = State."Wait for Event"  # Next State
            n102 = event-data() -> ()  [unwired: 1 in, 4 out]
            n103 = Unbundle By Name(w237) -> ("Device1 ID"=w236:dbl)
            n104 = call "Set DDS Amplitude Mv.vi"("amplitdude"="DDS1 Amplitude", "channel_index"=0 ("y"), "dev_id"=w236) -> ()  [unwired: 8 in, 1 out]
          }
          event "DDS1 Bias": Value Change {
            w246 = State."Wait for Event"  # Next State
            n105 = event-data() -> ()  [unwired: 1 in, 4 out]
            n106 = Unbundle By Name(w243) -> ("Device1 ID"=w242:dbl)
            n107 = call "Set DDS Bias Mv.vi"("bias"="DDS1 Bias", "channel_index"=0 ("y"), "dev_id"=w242) -> ()  [unwired: 8 in, 1 out]
          }
          event "DDS2 Wave Style": Value Change {
            w251 = State."Wait for Event"  # Next State
            # "W_SINE = 0x0001, \n\t\t\t\t\t\tW_SQUARE = 0x0002, \n\t\t\t\t\t\tW_RAMP = 0x0004, \n\t\t\t\t\t\tW_PULSE = 0x0008, \n\t\t\t\t\t\tW_NOISE = 0x0010, \n\t\t\t\t\t\tW_DC = 0x0020, \n\t\t\t\t\t\tW_ARB = 0x0040"
            n108 = event-data() -> ()  [unwired: 1 in, 4 out]
            n109 = Unbundle By Name(w249) -> ("Device1 ID"=w248:dbl)
            n110 = case shown="2" "DDS2 Wave Style" {
              tunnel: w248 -> [w253 w256 w259]
              frame 0, Default {
                n111 = call "Set DDS Boxing Style.vi"("boxing"=1 ("y"), "channel_index"=0 ("y"), "dev_id"=w253) -> ()  [unwired: 8 in, 1 out]
              }
              frame 1 {
                n112 = call "Set DDS Boxing Style.vi"("boxing"=2 ("y"), "channel_index"=0 ("y"), "dev_id"=w256) -> ()  [unwired: 8 in, 1 out]
              }
              frame 2 {
                n113 = call "Set DDS Boxing Style.vi"("boxing"=4 ("y"), "channel_index"=1 ("y"), "dev_id"=w259) -> ()  [unwired: 8 in, 1 out]
              }
            }
          }
          event "DDS2 Freq": Value Change {
            w266 = State."Wait for Event"  # Next State
            n114 = event-data() -> ()  [unwired: 1 in, 4 out]
            n115 = Unbundle By Name(w263) -> ("Device1 ID"=w262:dbl)
            n116 = call "Set DDS Freq.vi"("freq"="DDS2 Freq", "channel_index"=1 ("y"), "dev_id"=w262) -> ()  [unwired: 8 in, 1 out]
          }
          event "DDS2 Bias": Value Change {
            w271 = State."Wait for Event"  # Next State
            n117 = event-data() -> ()  [unwired: 1 in, 4 out]
            n118 = Unbundle By Name(w269) -> ("Device1 ID"=w268:dbl)
            n119 = call "Set DDS Bias Mv.vi"("bias"="DDS2 Bias", "channel_index"=1 ("y"), "dev_id"=w268) -> ()  [unwired: 8 in, 1 out]
          }
          event "DDS2 Amplitude": Value Change {
            w277 = State."Wait for Event"  # Next State
            n120 = event-data() -> ()  [unwired: 1 in, 4 out]
            n121 = Unbundle By Name(w274) -> ("Device1 ID"=w275:dbl)
            n122 = call "Set DDS Amplitude Mv.vi"("amplitdude"="DDS2 Amplitude", "channel_index"=0 ("y"), "dev_id"=w275) -> ()  [unwired: 8 in, 1 out]
          }
        }
      }
      frame "Read Voltage" {
        w283 = i8 0 ("channel")
        w301 = i8 0 ("channel")
        w327 = State."Exit"  # Next State
        w326 = State."Capture"  # Next State
        w332 = i8 0 ("channel")
        w304 = i8 1 ("channel")
        w316 = i8 0 ("channel")
        w341 = FALSE  # Stop Loop?
        n123 = Unbundle By Name(w299) -> ("Captue Length"=w338:dbl)
        n124 = Unbundle By Name(w299) -> ("Device2 ID"=w298:dbl)
        n125 = Multiply(x=w338, y=1024) -> (x*y=w284:dbl)
        n126 = Unbundle By Name(w299) -> ("Device1 ID"=w300:dbl)
        n127 = call "Read Voltage Datas.vi"("length"=w284, "error in (no error)"=w320, "channel"=w316, "dev_id"=w300) -> ("error out"=w330:errorcluster, "buffer out"=w323:dbl[], "function return"=→"ReadVoltageData Return":u32)  [unwired: 5 in]
        n128 = call "Read Voltage Datas.vi"("length"=w284, "error in (no error)"=w330, "channel"=w304, "dev_id"=w300) -> ("error out"=w329:errorcluster, "buffer out"=w306:dbl[])  [unwired: 5 in, 1 out]
        n129 = call "Read Voltage Datas.vi"("length"=w284, "error in (no error)"=w329, "channel"=i8 2, "dev_id"=w300) -> ("error out"=w328:errorcluster, "buffer out"=w335:dbl[])  [unwired: 5 in, 1 out]
        n130 = call "Read Voltage Datas.vi"("length"=w284, "error in (no error)"=w328, "channel"=i8 3, "dev_id"=w300) -> ("error out"=w293:errorcluster, "buffer out"=w334:dbl[])  [unwired: 5 in, 1 out]
        n131 = call "Read Voltage Datas.vi"("length"=w284, "error in (no error)"=w293, "channel"=i8 0, "dev_id"=w298) -> ("error out"=w292:errorcluster, "buffer out"=w289:dbl[])  [unwired: 5 in, 1 out]
        n132 = call "Read Voltage Datas.vi"("length"=w284, "error in (no error)"=w292, "channel"=i8 1, "dev_id"=w298) -> ("error out"=w291:errorcluster, "buffer out"=w288:dbl[])  [unwired: 5 in, 1 out]
        n133 = call "Read Voltage Datas.vi"("length"=w284, "error in (no error)"=w291, "channel"=i8 2, "dev_id"=w298) -> ("error out"=w290:errorcluster, "buffer out"=w287:dbl[])  [unwired: 5 in, 1 out]
        n134 = call "Read Voltage Datas.vi"("length"=w284, "error in (no error)"=w290, "channel"=i8 3, "dev_id"=w298) -> ("error out"=w281:errorcluster, "buffer out"=w286:dbl[])  [unwired: 5 in, 1 out]
        n135 = Build Array(w289, w288, w287, w286) -> (w285:dbl[][])
        n136 = Build Array(w323, w306, w335, w334) -> (w333:dbl[][])
        n137 = Array Subset(array=w285, index (row)=w283, length (row)=w284, index (col)=w283, length (col)=w284) -> (→"Voltage Wave":dbl[][])
        n138 = Array Subset(array=w333, index (row)=w332, length (row)=w284, index (col)=w332, length (col)=w284) -> (→"Voltage Wave":dbl[][])
        n139 = call "Get Osc Sample Rate.vi"("error in (no error)"=w281, "dev_id"=w300) -> ("error out"=w318:errorcluster, "function return"=w305:u32)  [unwired: 8 in]
        n140 = flat-sequence {
          tunnel: [w355] -> w310
          tunnel: w312 -> [w355]
          tunnel: w304 -> [w351]
          tunnel: w304 -> [w350]
          tunnel: [w354] -> w309
          tunnel: [w353] -> w308
          tunnel: [w352] -> w307
          tunnel: w300 -> [w349]
          frame #0 {
            n141 = call "Get Voltage Resolution.vi"("channel"=w351, "dev_id"=w349) -> ("function return"=w354:dbl)  [unwired: 8 in, 1 out]
            n142 = call "Get Voltage Extreme Max.vi"("channel"=w350, "dev_id"=w349) -> ("function return"=w353:dbl)  [unwired: 8 in, 1 out]
            n143 = call "Get Voltage Extreme Min.vi"("channel"=w350, "dev_id"=w349) -> ("function return"=w352:dbl)  [unwired: 8 in, 1 out]
          }
        }
        n144 = flat-sequence {
          tunnel: [w363] -> w317
          tunnel: w316 -> [w362]
          tunnel: [w361] -> w313
          tunnel: [w360] -> w314
          tunnel: w316 -> [w357]
          tunnel: [w359] -> w315
          tunnel: w316 -> [w358]
          tunnel: w318 -> [w363]
          tunnel: w300 -> [w356]
          frame #0 {
            n145 = call "Get Voltage Resolution.vi"("channel"=w358, "dev_id"=w356) -> ("function return"=w359:dbl)  [unwired: 8 in, 1 out]
            n146 = call "Get Voltage Extreme Max.vi"("channel"=w357, "dev_id"=w356) -> ("function return"=w360:dbl)  [unwired: 8 in, 1 out]
            n147 = call "Get Voltage Extreme Min.vi"("channel"=w362, "dev_id"=w356) -> ("function return"=w361:dbl)  [unwired: 8 in, 1 out]
          }
        }
        n148 = call "Para Cal Reset.vi"("para_chn"=w304, "voltage_resolution"=w309, "extreme_max"=w308, "buffer"=w306, "buffer_length"=w284, "sample"=w305, "error in (no error)"=w310, "extreme_min"=w307) -> ("function return"=w302:i32, "error out"=w311:errorcluster)  [unwired: 5 in, 1 out]
        n149 = call "Para Cal Reset.vi"("para_chn"=w316, "voltage_resolution"=w315, "extreme_max"=w314, "buffer"=w323, "buffer_length"=w284, "sample"=w305, "error in (no error)"=w317, "extreme_min"=w313) -> ("function return"=w321:i32, "error out"=w319:errorcluster)  [unwired: 5 in, 1 out]
        n150 = Equal?(x=w321, y=w301) -> (x = y?=w322:bool)
        n151 = Equal?(x=w301, y=w302) -> (x = y?=w303:bool)
        n152 = case shown="True" w322 {
          tunnel: w316 -> [_ w370]
          tunnel: [w364 w365] -> w312
          tunnel: w319 -> [w364 w365]
          frame False {
          }
          frame True {
            n153 = call "Get Min.vi"("para_chn"=w370) -> ("function return"=→"CH1 Min":dbl)  [unwired: 9 in, 1 out]
            n154 = call "Get Max.vi"("para_chn"=w370) -> ("function return"=→"CH1 Max":dbl)  [unwired: 9 in, 1 out]
            n155 = call "Get Vpp.vi"("para_chn"=w370) -> ("function return"=→"CH1 Vpp":dbl)  [unwired: 9 in, 1 out]
            n156 = call "Get Freq.vi"("para_chn"=w370) -> ("function return"=→"CH1 Frequency":dbl)  [unwired: 9 in, 1 out]
          }
        }
        n157 = case shown="True" w303 {
          tunnel: w304 -> [_ w348]
          tunnel: [w342 w343] -> w280
          tunnel: w311 -> [w342 w343]
          frame False {
          }
          frame True {
            n158 = call "Get Min.vi"("para_chn"=w348) -> ("function return"=→"CH2 Min":dbl)  [unwired: 9 in, 1 out]
            n159 = call "Get Max.vi"("para_chn"=w348) -> ("function return"=→"CH2 Max":dbl)  [unwired: 9 in, 1 out]
            n160 = call "Get Vpp.vi"("para_chn"=w348) -> ("function return"=→"CH2 Vpp":dbl)  [unwired: 9 in, 1 out]
            n161 = call "Get Freq.vi"("para_chn"=w348) -> ("function return"=→"CH2 Frequency":dbl)  [unwired: 9 in, 1 out]
          }
        }
        n162 = Unbundle By Name(w299) -> ("Boolean <Is Exit>"=w324:bool)
        n163 = Select(t=w327, s=w324, f=w326) -> (s? t:f=w325:T2)
      }
      frame "Read IO" {
        w374 = FALSE  # Stop Loop?
        w375 = State."Wait for Event"  # Next State
        w381 = 16 ("front")
        w378 = 1 ("front")
        n164 = Unbundle By Name(w373) -> ("Device1 ID"=w372:dbl)
        n165 = call "Get IO In State.vi"("dev_id"=w372) -> ("function return"=w377:u32)  [unwired: 9 in, 1 out]
        "IO Read Return" <- w377
        n166 = And(x=w377, y=w381) -> (x .and. y?=w380:u32)
        n167 = And(x=w377, y=w378) -> (x .and. y?=w376:u32)
        n168 = Equal?(x=w376, y=w378) -> (x = y?=→"IO0":bool)
        n169 = Equal?(x=w380, y=w381) -> (x = y?=→"IO4":bool)
      }
      frame "Exit" {
        w388 = TRUE  # Stop Loop?
        w389 = State."Exit"  # (Value Not Used)
        # "#CodeNeeded - Add any required cleanup code here."
        # "The state value is not used here since this is the last iteration of the state machine loop."
        # "Exit - Exit the application."
        n170 = flat-sequence {
          tunnel: [w392] -> w387
          tunnel: w385 -> [w390]
          tunnel: [w390] -> w384
          tunnel: w387 -> [w399]
          tunnel: w384 -> [w397]
          frame #0 {
            w393 = i8 16  # IO Num
            w392 = i8 0  # en
            n171 = for {
              N: w393 -> [_]
              tunnel: w392 -> [w395]
              tunnel: w390 -> [w394]
              i -> [w396]
              n172 = call "IO Enable.vi"("enable"=w395, "channel"=w396, "dev_id"=w394) -> ()  [unwired: 8 in, 1 out]
            }
            n173 = Wait (ms)(milliseconds to wait=1000) -> ()  [unwired: 1 out]
          }
          frame #1 {
            w401 = i8 1  # channel
            w400 = i8 0  # channel
            n174 = call "DDS Output Enable.vi"("enable"=w399, "channel_index"=w400, "dev_id"=w397) -> ("error out"=w402:errorcluster)  [unwired: 8 in]
            n175 = call "DDS Output Enable.vi"("error in (no error)"=w402, "enable"=w399, "channel_index"=w401, "dev_id"=w397) -> ()  [unwired: 7 in, 1 out]
            n176 = Wait (ms)(milliseconds to wait=1000) -> ()  [unwired: 1 out]
          }
          frame #2 {
            n177 = call "Finish Dll.vi"() -> ()  [unwired: 10 in, 2 out]
          }
        }
        n178 = Unbundle By Name(w386) -> ("Device1 ID"=w385:dbl)
      }
    }
    n179 = Or(x=w6, y=w7) -> (x .or. y?=w8:bool)
  }
  n180 = call <vilib>:"Simple Error Handler.vi"("error in (no error)"=w2) -> ("error out"=w1:errorcluster)  [unwired: 4 in, 4 out]
  n181 = disable-structure shown="RUN_TIME_ENGINE==True" {
    disable-tunnel: w1 -> [_ _]
    frame condition #0 (active) {
    }
    frame condition #1 {
      # "Call Quit LabVIEW if running as a built application."
      n182 = Quit LabVIEW() -> ()  [unwired: 1 in]
    }
  }
